vi "Wait For Temperature.vi"(4 "error in (no error)":errorcluster, 6 "Delay (s)":u32=5, 7 "Instrument Ref In":refnum<k24>) -> (0 "error out":errorcluster, 1 "Temperature\nStatus":i32(ring) items=["TemperatureUnknown"=0, "Stable"=1, "Tracking"=2, "Near"=5, "Chasing"=6, "Filling"=7, "Standby"=10, "Disabled"=13, "ImpedanceNotFunction"=14, "TempFailure"=15], 2 "Temperature":dbl, 3 "Instrument Ref Out":refnum<k24>)   [LabVIEW 2020]
uses:
  C:/Users/qmgmit/Desktop/Shivam/dev/QDInstrument/QDInstrument.dll
  dev/QDInstrument/QDInstrument.dll
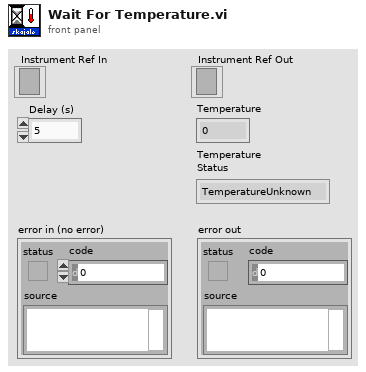
[diagram p1: front panel]
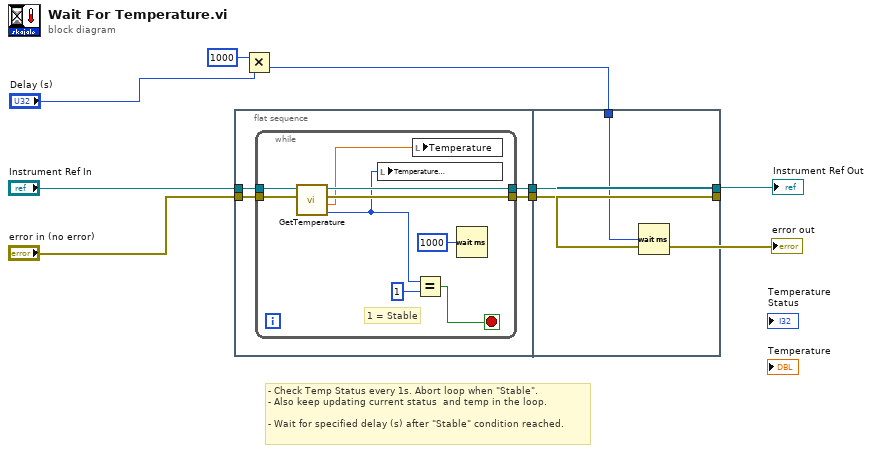
[diagram p0: block diagram]
diagram:
  # "- Check Temp Status every 1s. Abort loop when \"Stable\".\n- Also keep updating current status  and temp in the loop.\n\n- Wait for specified delay (s) after \"Stable\" condition reached."
  n1 = flat-sequence {
    tunnel: "Instrument Ref In" -> [w13]
    tunnel: "error in (no error)" -> [w11]
    tunnel: [w12] -> w5
    tunnel: [w10] -> w4
    tunnel: [w24] -> w6
    tunnel: [w25] -> w8
    tunnel: w5 -> [w25]
    tunnel: w4 -> [w24]
    tunnel: w2 -> [w23]
    frame #0 {
      n2 = while {
        tunnel: w13 -> [w22]
        tunnel: [w21] -> w12
        tunnel: w11 -> [w20]
        tunnel: [w19] -> w10
        stop <- w17 stop-if-true
        # "1 = Stable"
        n3 = call <userlib>:"GetTemperature.vi"("error in (no error)"=w20, "Instrument Ref In"=w22) -> ("Temperature\nStatus"=w14:i32, "Temperature"=w15:dbl, "error out"=w19:errorcluster, "Instrument Ref Out"=w21:refnum<k24>)  [unwired: 3 in, 1 out]
        n4 = local write "Temperature\nStatus"(w14) -> ()
        n5 = local write "Temperature"(w15) -> ()
        n6 = Equal?(x=w14, y=1) -> (x = y?=w17:bool)
        n7 = Wait (ms)(milliseconds to wait=u32 1000) -> ()  [unwired: 1 out]
      }
    }
    frame #1 {
      n8 = Wait (ms)(milliseconds to wait=w23) -> ()  [unwired: 1 out]
    }
  }
  n9 = Multiply(x=u32 1000, y="Delay (s)") -> (x*y=w2:u32)
  "Instrument Ref Out" <- w8
  "error out" <- w6
